vi "Update State.vi"(8 "error in (no error)":errorcluster, 10 "State":T1, 11 "Module in":refnum<class "Module.lvclass">) -> (0 "error out":errorcluster, 3 "Module out":refnum<class "Module.lvclass">)   [LabVIEW 2020, in "Volatus.lvlib" / "Module.lvclass"]
uses:
  Module.lvclass
  State.ctl
  Module Status.ctl
  MessageQ/MessageQ.lvclass
  Event Level.ctl
  Module.lvclass/Module.ctl
  MessageQ/MessageQ.lvclass/MessageQ.ctl
  Volatus.lvlib
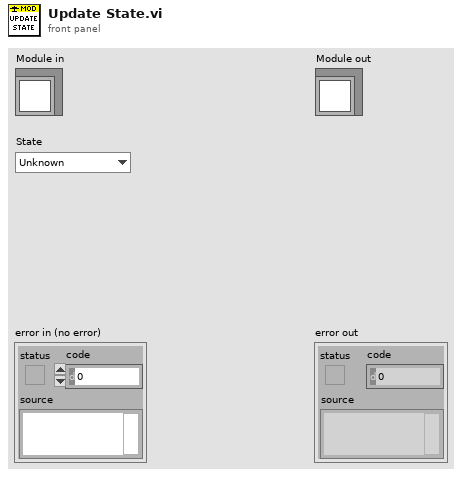
[diagram p1: front panel]
types:
  T1 = typedef "Volatus.lvlib/Module.lvclass/State.ctl" = enum16{"Unknown", "Launched", "Starting", "Running", "Stopping", "Stopped", "Error - Starting", "Error - Run", "Error - Stopping"}
  T2 = typedef "Volatus.lvlib/Event Level.ctl" = enum16{"Debug", "Info", "Warning", "Error"}
  T3 = typedef "Volatus.lvlib/Module Status.ctl" = cluster{"MessageQ":refnum<class "MessageQ.lvclass">, "State":T1, "Hierarchy":string[]}
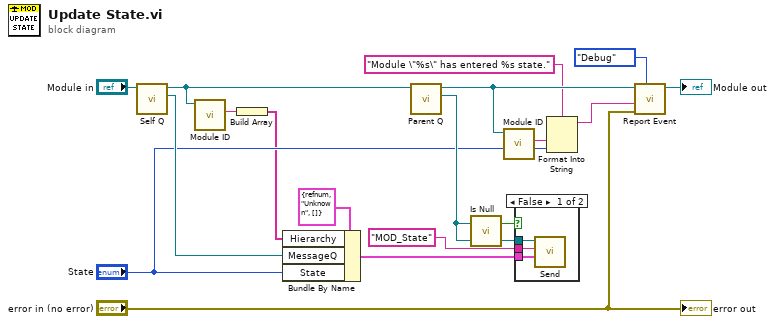
[diagram p0: block diagram]
diagram:
  n1 = call "Self Q.vi"("Module in"="Module in") -> ("Self Q"=w14:refnum<class "MessageQ.lvclass">, "Module out"=w3:refnum<class "Module.lvclass">)  [unwired: 9 in]
  n2 = call-dynamic "Module ID.vi"("Module in"=w3) -> ("Module ID"=w2:string)  [unwired: 10 in]
  n3 = Build Array(w2) -> (w1:string[])
  n4 = Bundle By Name(cluster=T3 {"MessageQ"=refnum, "State"=enum."Unknown", "Hierarchy"=[]} ("Nested State Data"), "Hierarchy"=w1, "MessageQ"=w14, "State"="State") -> (w15:T3)
  n5 = call "Parent Q.vi"("Module in"=w3) -> ("Parent Q"=w13:refnum<class "MessageQ.lvclass">, "Module out"=w9:refnum<class "Module.lvclass">)  [unwired: 9 in]
  n6 = call "Is Null.vi"("MessageQ in"=w13) -> ("Null"=w12:bool)  [unwired: 2 in]
  n7 = call-dynamic "Module ID.vi"("Module in"=w9) -> ("Module ID"=w7:string)  [unwired: 10 in]
  n8 = case shown="False" w12 {
    tunnel: "MOD_State" ("ID") -> [w21 _]
    tunnel: w15 -> [w20 _]
    tunnel: w13 -> [w19 _]
    frame False {
      n9 = call "Send.vi"("Data"=w20, "ID"=w21, "MessageQ in"=w19) -> ()  [unwired: 7 in, 2 out]
    }
    frame True {
    }
  }
  n10 = Format Into String(format string="Module \"%s\" has entered %s state.", w7, "State") -> (resulting string=w5:string)  [unwired: 2 in, 1 out]
  n11 = call "Report Event.vi"("Level (Info)"=Event_Level."Debug", "error in (no error)"="error in (no error)", "Message"=w5, "Module in"=w9) -> ("Module out"=→"Module out":refnum<class "Module.lvclass">)  [unwired: 6 in, 1 out]
  "error out" <- "error in (no error)"
